vi "Camera_acquisition_test.vi"() -> ()   [LabVIEW 2024]
panel:
  in  "ICImagingControl":refnum<k7>(container)
  in  "Open Device Configuration (Monochrome  Images)":bool
  in  "Open Device Configuration (Color Images)":bool
  in  "Grab":bool
  in  "End Program":bool
  # "Open Device Configuration"
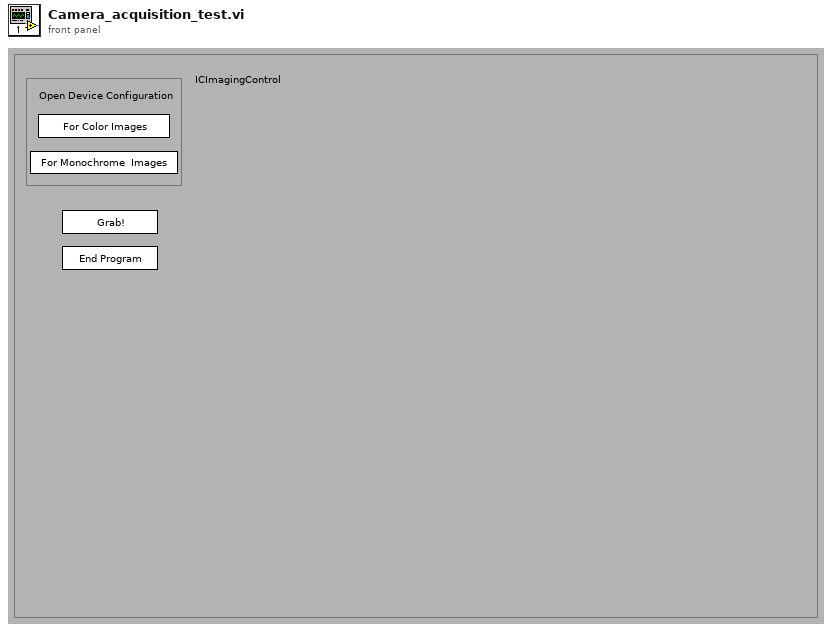
[diagram p1: front panel]
types:
  T1 = typedef "IMAQ Image.ctl" = refnum<image>
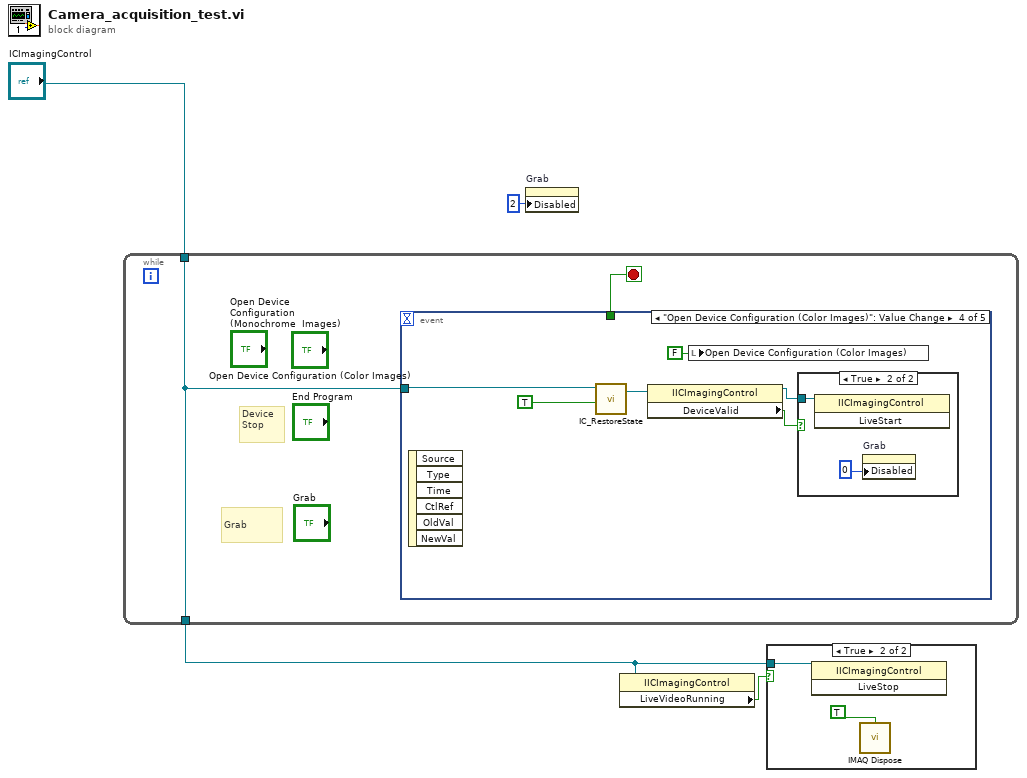
[diagram p0: block diagram]
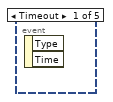
[diagram p3: hidden frame]
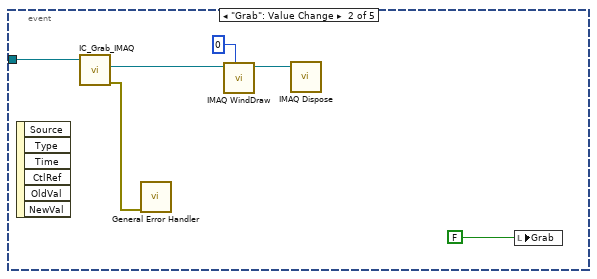
[diagram p4: hidden frame]
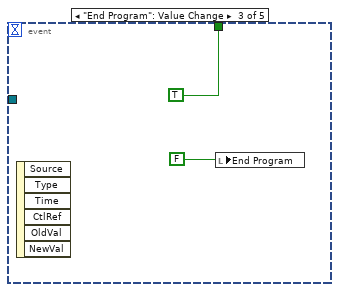
[diagram p5: hidden frame]
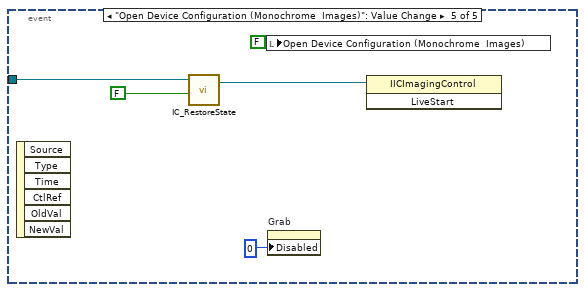
[diagram p7: hidden frame]
diagram:
  n1 = while {
    tunnel: "ICImagingControl" -> [w5]
    tunnel: [w5] -> w3
    stop <- w6 stop-if-true
    # "Device\nStop"
    # "Grab"
    n2 = event shown="[3] \"Open Device Configuration (Color Images)\": Value Change" {
      selector: _ -> [_ _ _ _ _]
      dyn-events: _ -> [_ _ _ _ _]
      timeout: _ -> [_ _ _ _ _]
      tunnel: w5 -> [_ w11 _ w18 w23]
      tunnel: [_ _ TRUE _ _] -> w6
      event Timeout {
        n3 = event-data() -> ()  [unwired: 1 in, 2 out]
      }
      event "Grab": Value Change {
        n4 = event-data() -> ()  [unwired: 1 in, 6 out]
        n5 = call <userlib>:"IC_Grab_IMAQ.vi"("ICImagingControl In"=w11) -> ("Image Out"=w9:T1, "Error Out"=w10:errorcluster)  [unwired: 2 in, 2 out]
        n6 = call <vilib>:"General Error Handler.vi"("error in (no error)"=w10) -> ()  [unwired: 10 in, 5 out]
        n7 = call "IMAQ WindDraw"("Window Number (0...15)"=0, "Image"=w9) -> ("Image Out (duplicate)"=w7:T1)  [unwired: 8 in, 1 out]
        n8 = call "IMAQ Dispose"("Image"=w7) -> ()  [unwired: 5 in, 1 out]
        n9 = local write "Grab"(FALSE) -> ()
      }
      event "End Program": Value Change {
        n10 = event-data() -> ()  [unwired: 1 in, 6 out]
        n11 = local write "End Program"(FALSE) -> ()
      }
      event "Open Device Configuration (Color Images)": Value Change {
        n12 = event-data() -> ()  [unwired: 1 in, 6 out]
        n13 = call <userlib>:"IC_RestoreState.vi"("Color"=TRUE, "ICImagingControl"=w18) -> ("ICImagingControl Out"=w17:refnum<k7>)  [unwired: 2 in, 1 out]
        n14 = property class="IICImagingControl"(reference=w17) -> (reference out=w15:refnum<k7>, "DeviceValid"=w16:bool)  [unwired: 1 in, 1 out]
        n15 = local write "Open Device Configuration (Color Images)"(FALSE ("Open Device Configuration (Color Images)")) -> ()
        n16 = case shown="True" w16 {
          tunnel: w15 -> [_ w22]
          frame False {
          }
          frame True {
            n17 = invoke class="IICImagingControl" method="LiveStart"(reference=w22) -> ()  [unwired: 2 in, 3 out]
            n18 = property on="Grab" class="Bool (strict)"("Disabled"=u8 0) -> ()  [unwired: 2 in, 2 out]
          }
        }
      }
      event "Open Device Configuration (Monochrome  Images)": Value Change {
        n19 = event-data() -> ()  [unwired: 1 in, 6 out]
        n20 = call <userlib>:"IC_RestoreState.vi"("Color"=FALSE, "ICImagingControl"=w23) -> ("ICImagingControl Out"=w26:refnum<k7>)  [unwired: 2 in, 1 out]
        n21 = local write "Open Device Configuration (Monochrome  Images)"(FALSE) -> ()
        n22 = property on="Grab" class="Bool (strict)"("Disabled"=0) -> ()  [unwired: 2 in, 2 out]
        n23 = invoke class="IICImagingControl" method="LiveStart"(reference=w26) -> ()  [unwired: 2 in, 3 out]
      }
    }
  }
  n24 = property on="Grab" class="Bool (strict)"("Disabled"=u8 2) -> ()  [unwired: 2 in, 2 out]
  n25 = property class="IICImagingControl"(reference=w3) -> ("LiveVideoRunning"=w4:bool)  [unwired: 1 in, 2 out]
  n26 = case shown="True" w4 {
    tunnel: w3 -> [_ w29]
    frame False {
    }
    frame True {
      n27 = invoke class="IICImagingControl" method="LiveStop"(reference=w29) -> ()  [unwired: 2 in, 3 out]
      n28 = call "IMAQ Dispose"("All Images? (No)"=TRUE) -> ()  [unwired: 5 in, 1 out]
    }
  }
